vi "Test REF Configuration.vi"(8 "error in (no error)":errorcluster, 11 "Instrument.Lockin in":refnum<class "Instrument.Lockin.lvclass">) -> (0 "error out":errorcluster, 3 "Instrument.Lockin out":refnum<class "Instrument.Lockin.lvclass">)   [LabVIEW 2019]
uses:
  src/Instrument.Lockin/Instrument.Lockin.lvclass
  <vilib>/addons/_JKI Toolkits/Caraya/classes/Assert/Assert Equal Value and Type_Variant.vi
  <userlib>/_OpenG.lib/numeric/numeric.llb/Random Number Within Range - DBL__ogtk.vi
  <vilib>/addons/_JKI Toolkits/Caraya/classes/Assert/Assert Almost Equal_Float.vi
  <userlib>/_OpenG.lib/numeric/numeric.llb/Random Number Within Range - I32__ogtk.vi
  <vilib>/addons/_JKI Toolkits/Caraya/classes/Test/Test.lvclass
  <vilib>/addons/_JKI Toolkits/Caraya/classes/Assert/Assert.lvclass
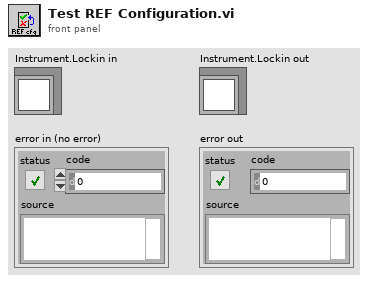
[diagram p1: front panel]
types:
  T1 = typedef "Instrument.Lockin.lvlib/Instrument.DAQ.lvclass/REF.Channel--Cluster--Array.ctl" = T2[]
  T2 = typedef "Instrument.Lockin.lvlib/Instrument.DAQ.lvclass/REF.Channel--Cluster.ctl" = cluster{"Enable?":bool, "Channel":i32, "Frequency":dbl, "Phase":dbl, "TC":dbl, "Roll-Off":i32}
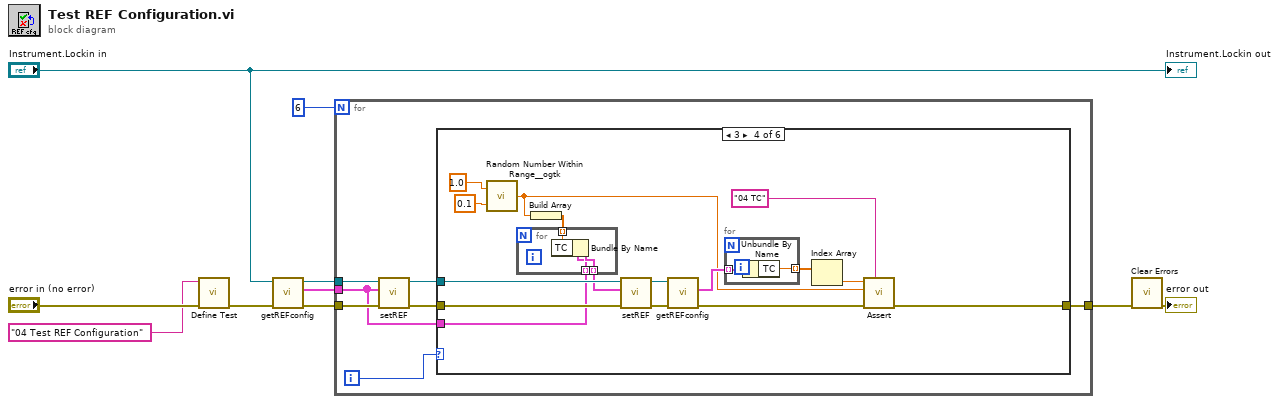
[diagram p0: block diagram]
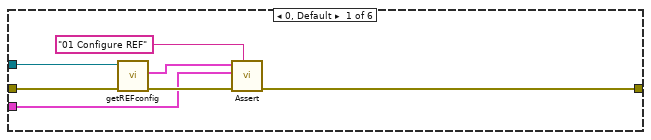
[diagram p2: hidden frame]
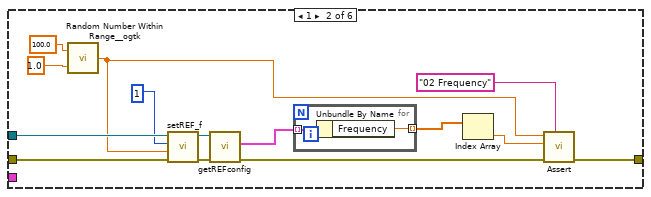
[diagram p3: hidden frame]
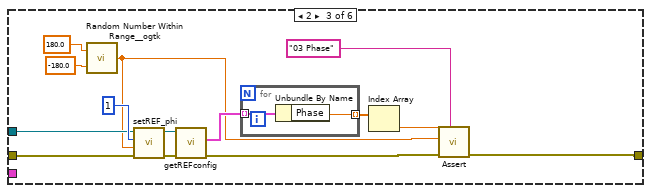
[diagram p4: hidden frame]
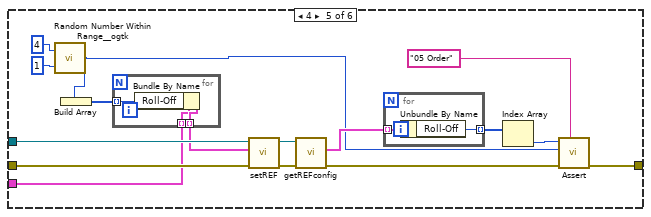
[diagram p5: hidden frame]
diagram:
  n1 = call <vilib>:"Define Test.vi"("error in (no error)"="error in (no error)", "Label (VI Title)"="04 Test REF Configuration") -> ("error out"=w2:errorcluster)  [unwired: 8 in, 1 out]
  n2 = call-dynamic "getREFconfig.vi"("error in (no error)"=w2, "Instrument.Lockin in"="Instrument.Lockin in") -> ("error out"=w1:errorcluster, "REFconfig"=w3:T1, "Instrument.Lockin out"=w4:refnum<class "Instrument.Lockin.lvclass">)  [unwired: 7 in]
  n3 = for {
    N: 6 -> [_]
    tunnel: w1 -> [w16]
    tunnel: w4 -> [w15]
    tunnel: w3 -> [w12]
    tunnel: [w11] -> w6
    i -> [w17]
    n4 = call-dynamic "setREF.vi"("error in (no error)"=w16, "Channels: Lockin in"=w12, "Instrument.Lockin in"=w15) -> ("error out"=w14:errorcluster, "Instrument.Lockin out"=w13:refnum<class "Instrument.Lockin.lvclass">)  [unwired: 7 in]
    n5 = case shown="3" w17 {
      tunnel: w14 -> [w22 w31 w47 w65 w88 w99]
      tunnel: w13 -> [w21 w30 w46 w66 w89 _]
      tunnel: w12 -> [w20 _ _ w59 w83 _]
      tunnel: [w18 w25 w41 w57 w78 w99] -> w11
      frame 0, Default {
        n6 = call-dynamic "getREFconfig.vi"("error in (no error)"=w22, "Instrument.Lockin in"=w21) -> ("error out"=w23:errorcluster, "REFconfig"=w19:T1)  [unwired: 7 in, 1 out]
        n7 = call-poly <vilib>:"Assert.vi"("Label"="01 Configure REF", "error in (no error)"=w23, "Actual"=w20, "Expected"=w19) -> ("error out"=w18:errorcluster)  [unwired: 6 in, 1 out]
      }
      frame 1 {
        n8 = call-poly <userlib>:"Random Number Within Range__ogtk.vi"("High"=100.0, "Low"=1.0) -> ("Random Number"=w27:dbl)  [unwired: 3 in]
        n9 = call-dynamic "setREF_f.vi"("error in (no error)"=w31, "Frequency (Hz)"=w27, "REF Channel"=1, "Instrument.Lockin in"=w30) -> ("error out"=w32:errorcluster, "Instrument.Lockin out"=w33:refnum<class "Instrument.Lockin.lvclass">)  [unwired: 6 in]
        n10 = call-dynamic "getREFconfig.vi"("error in (no error)"=w32, "Instrument.Lockin in"=w33) -> ("error out"=w36:errorcluster, "REFconfig"=w26:T1)  [unwired: 7 in, 1 out]
        n11 = for {
          tunnel: [w40] -> w37 mode=indexing
          tunnel: w26 -> [w39] mode=indexing
          n12 = Unbundle By Name(w39) -> ("Frequency"=w40:dbl)
        }
        n13 = Index Array(array=w37) -> (element=w28:dbl)  [unwired: 1 in]
        n14 = call-poly <vilib>:"Assert.vi"("Label"="02 Frequency", "error in (no error)"=w36, "Actual"=w28, "Expected"=w27) -> ("error out"=w25:errorcluster)  [unwired: 6 in, 1 out]
      }
      frame 2 {
        n15 = call-poly <userlib>:"Random Number Within Range__ogtk.vi"("High"=180.0, "Low"=-180.0) -> ("Random Number"=w42:dbl)  [unwired: 3 in]
        n16 = call-dynamic "setREF_phi.vi"("error in (no error)"=w47, "Phase (°)"=w42, "REF Channel"=1, "Instrument.Lockin in"=w46) -> ("error out"=w48:errorcluster, "Instrument.Lockin out"=w49:refnum<class "Instrument.Lockin.lvclass">)  [unwired: 6 in]
        n17 = call-dynamic "getREFconfig.vi"("error in (no error)"=w48, "Instrument.Lockin in"=w49) -> ("error out"=w45:errorcluster, "REFconfig"=w54:T1)  [unwired: 7 in, 1 out]
        n18 = for {
          tunnel: w54 -> [w56] mode=indexing
          tunnel: [w55] -> w53 mode=indexing
          n19 = Unbundle By Name(w56) -> ("Phase"=w55:dbl)
        }
        n20 = Index Array(array=w53) -> (element=w43:dbl)  [unwired: 1 in]
        n21 = call-poly <vilib>:"Assert.vi"("Label"="03 Phase", "error in (no error)"=w45, "Actual"=w42, "Expected"=w43) -> ("error out"=w41:errorcluster)  [unwired: 6 in, 1 out]
      }
      frame 3 {
        n22 = call-poly <userlib>:"Random Number Within Range__ogtk.vi"("High"=1.0, "Low"=0.1) -> ("Random Number"=w58:dbl)  [unwired: 3 in]
        n23 = Build Array(w58) -> (w63:dbl[])
        n24 = for {
          tunnel: [w75] -> w64 mode=indexing
          tunnel: w63 -> [w74] mode=indexing
          tunnel: w59 -> [w73] mode=indexing
          n25 = Bundle By Name(cluster=w73, "TC"=w74) -> (w75:T2)
        }
        n26 = call-dynamic "setREF.vi"("error in (no error)"=w65, "Channels: Lockin in"=w64, "Instrument.Lockin in"=w66) -> ("error out"=w68:errorcluster, "Instrument.Lockin out"=w67:refnum<class "Instrument.Lockin.lvclass">)  [unwired: 7 in]
        n27 = call-dynamic "getREFconfig.vi"("error in (no error)"=w68, "Instrument.Lockin in"=w67) -> ("error out"=w60:errorcluster, "REFconfig"=w72:T1)  [unwired: 7 in, 1 out]
        n28 = for {
          tunnel: w72 -> [w77] mode=indexing
          tunnel: [w76] -> w71 mode=indexing
          n29 = Unbundle By Name(w77) -> ("TC"=w76:dbl)
        }
        n30 = Index Array(array=w71) -> (element=w61:dbl)  [unwired: 1 in]
        n31 = call-poly <vilib>:"Assert.vi"("Label"="04 TC", "error in (no error)"=w60, "Actual"=w58, "Expected"=w61) -> ("error out"=w57:errorcluster)  [unwired: 6 in, 1 out]
      }
      frame 4 {
        n32 = call-poly <userlib>:"Random Number Within Range__ogtk.vi"("High"=4, "Low"=1) -> ("Random Number"=w81:i32)  [unwired: 3 in]
        n33 = Build Array(w81) -> (w86:i32[])
        n34 = for {
          tunnel: [w96] -> w87 mode=indexing
          tunnel: w86 -> [w95] mode=indexing
          tunnel: w83 -> [w94] mode=indexing
          n35 = Bundle By Name(cluster=w94, "Roll-Off"=w95) -> (w96:T2)
        }
        n36 = call-dynamic "setREF.vi"("error in (no error)"=w88, "Channels: Lockin in"=w87, "Instrument.Lockin in"=w89) -> ("error out"=w91:errorcluster, "Instrument.Lockin out"=w90:refnum<class "Instrument.Lockin.lvclass">)  [unwired: 7 in]
        n37 = call-dynamic "getREFconfig.vi"("error in (no error)"=w91, "Instrument.Lockin in"=w90) -> ("error out"=w80:errorcluster, "REFconfig"=w93:T1)  [unwired: 7 in, 1 out]
        n38 = for {
          tunnel: w93 -> [w98] mode=indexing
          tunnel: [w97] -> w92 mode=indexing
          n39 = Unbundle By Name(w98) -> ("Roll-Off"=w97:i32)
        }
        n40 = Index Array(array=w92) -> (element=w82:i32)  [unwired: 1 in]
        n41 = call-poly <vilib>:"Assert.vi"("Label"="05 Order", "error in (no error)"=w80, "Actual"=w81, "Expected"=w82) -> ("error out"=w78:errorcluster)  [unwired: 6 in, 1 out]
      }
      frame 5 {
      }
    }
  }
  n42 = call <vilib>:"Clear Errors.vi"("error in (no error)"=w6) -> ("error out"=→"error out":errorcluster)  [unwired: 5 in, 1 out]
  "Instrument.Lockin out" <- "Instrument.Lockin in"
